vi "Create Notifiers.vi"(8 "error in":errorcluster) -> (0 "error out":errorcluster, 3 "Notifiers":T1)   [LabVIEW 2014]
uses:
  Notifiers.ctl
  Message Handler Loop Notifiers.ctl
  Hardware Control/Parameter Analyzer/Parameter Analyzer Notifiers.ctl
  Hardware Control/Switching Matrix/Switching Matrix Notifiers.ctl
  Hardware Control/Stress Control/StressControl Notifiers.ctl
  Hardware Control/Spectrometer/Spectrometer Notifiers.ctl
  Hardware Control/Switches and Mirrors/SwitchesMirrors Notifiers.ctl
  Hardware Control/Camera/Camera Notifiers.ctl
  Hardware Control/XYZ Stage/XYZ Notifications.ctl
  Hardware Control/Autofocus/Autofocus Notifiers.ctl
  Measurements/Optoelectronic Measurement/Optoelectronic Notifiers.ctl
  Measurements/Save Data/SaveData Notifiers.ctl
  Measurements/Instrument Sequence/Instrument Sequence Notifiers.ctl
panel:
  # "LICENSED MATERIALS – PROPERTY OF IBM\nCopyright IBM Corp. 2016,\nALL RIGHTS RESERVED"
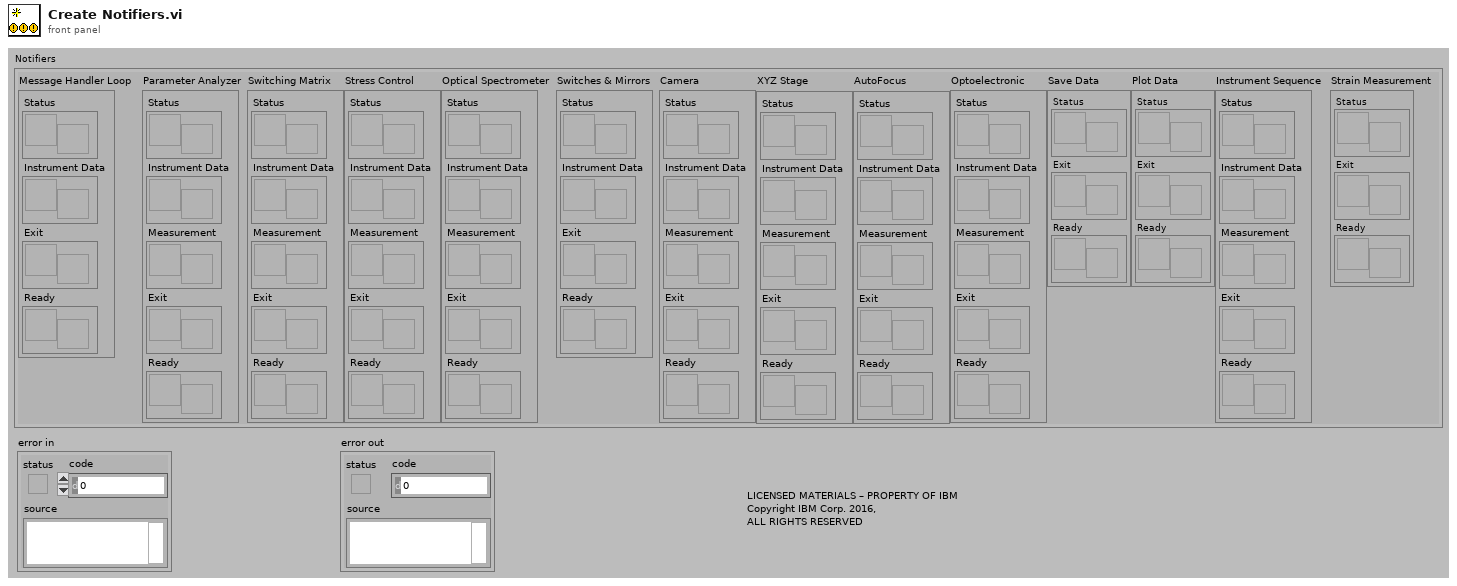
[diagram p1: front panel]
types:
  T1 = typedef "Notifiers.ctl" = cluster{"Message Handler Loop":T2, "Parameter Analyzer":T3, "Switching Matrix":T4, "Stress Control":T5, "Optical Spectrometer":T6, "Switches & Mirrors":T7, "Camera":T8, "XYZ Stage":T9, "AutoFocus":T10, "Optoelectronic":T11, "Save Data":T12, "Plot Data":T12, "Instrument Sequence":T13, "Strain Measurement":cluster{"Status":refnum<notifier>, "Exit":refnum<notifier>, "Ready":refnum<notifier>}}
  T2 = typedef "Message Handler Loop Notifiers.ctl" = cluster{"Status":refnum<notifier>, "Instrument Data":refnum<notifier>, "Exit":refnum<notifier>, "Ready":refnum<notifier>}
  T3 = typedef "Parameter Analyzer Notifiers.ctl" = cluster{"Status":refnum<notifier>, "Instrument Data":refnum<notifier>, "Measurement":refnum<notifier>, "Exit":refnum<notifier>, "Ready":refnum<notifier>}
  T4 = typedef "Switching Matrix Notifiers.ctl" = cluster{"Status":refnum<notifier>, "Instrument Data":refnum<notifier>, "Measurement":refnum<notifier>, "Exit":refnum<notifier>, "Ready":refnum<notifier>}
  T5 = typedef "StressControl Notifiers.ctl" = cluster{"Status":refnum<notifier>, "Instrument Data":refnum<notifier>, "Measurement":refnum<notifier>, "Exit":refnum<notifier>, "Ready":refnum<notifier>}
  T6 = typedef "Spectrometer Notifiers.ctl" = cluster{"Status":refnum<notifier>, "Instrument Data":refnum<notifier>, "Measurement":refnum<notifier>, "Exit":refnum<notifier>, "Ready":refnum<notifier>}
  T7 = typedef "SwitchesMirrors Notifiers.ctl" = cluster{"Status":refnum<notifier>, "Instrument Data":refnum<notifier>, "Exit":refnum<notifier>, "Ready":refnum<notifier>}
  T8 = typedef "Camera Notifiers.ctl" = cluster{"Status":refnum<notifier>, "Instrument Data":refnum<notifier>, "Measurement":refnum<notifier>, "Exit":refnum<notifier>, "Ready":refnum<notifier>}
  T9 = typedef "XYZ Notifications.ctl" = cluster{"Status":refnum<notifier>, "Instrument Data":refnum<notifier>, "Measurement":refnum<notifier>, "Exit":refnum<notifier>, "Ready":refnum<notifier>}
  T10 = typedef "Autofocus Notifiers.ctl" = cluster{"Status":refnum<notifier>, "Instrument Data":refnum<notifier>, "Measurement":refnum<notifier>, "Exit":refnum<notifier>, "Ready":refnum<notifier>}
  T11 = typedef "Optoelectronic Notifiers.ctl" = cluster{"Status":refnum<notifier>, "Instrument Data":refnum<notifier>, "Measurement":refnum<notifier>, "Exit":refnum<notifier>, "Ready":refnum<notifier>}
  T12 = typedef "SaveData Notifiers.ctl" = cluster{"Status":refnum<notifier>, "Exit":refnum<notifier>, "Ready":refnum<notifier>}
  T13 = typedef "Instrument Sequence Notifiers.ctl" = cluster{"Status":refnum<notifier>, "Instrument Data":refnum<notifier>, "Measurement":refnum<notifier>, "Exit":refnum<notifier>, "Ready":refnum<notifier>}
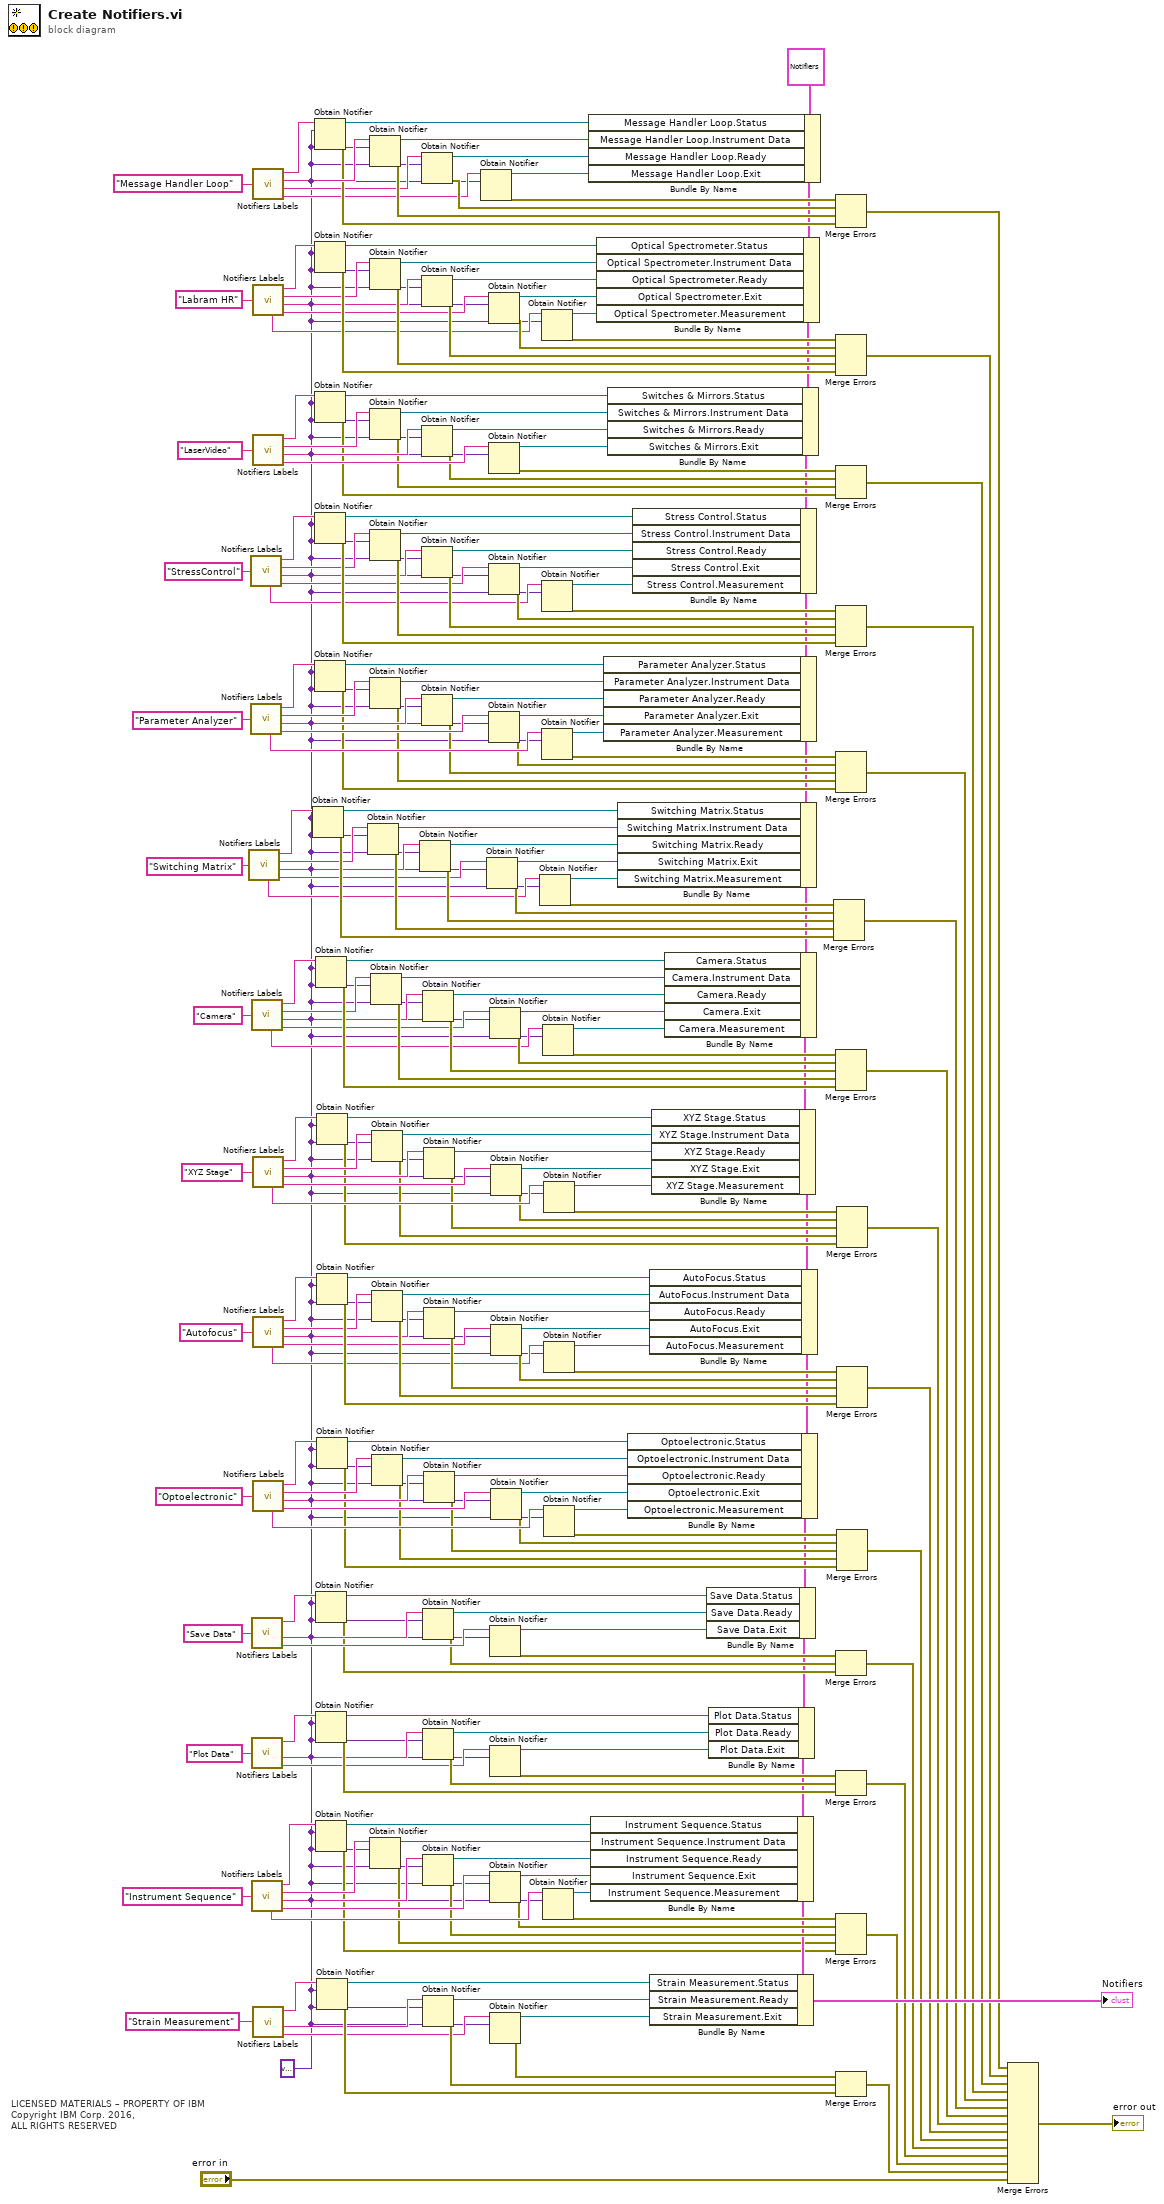
[diagram p0: block diagram]
diagram:
  w1 = variant ("element data type")
  # "LICENSED MATERIALS – PROPERTY OF IBM\nCopyright IBM Corp. 2016,\nALL RIGHTS RESERVED"
  n1 = call "Notifiers Labels.vi"("Instrument"="Switching Matrix") -> ("Exit String"=w117:string, "Ready String"=w118:string, "Data String"=w119:string, "Status String"=w120:string, "Measurement String"=w116:string)
  n2 = call "Notifiers Labels.vi"("Instrument"="StressControl") -> ("Exit String"=w185:string, "Ready String"=w186:string, "Data String"=w187:string, "Status String"=w188:string, "Measurement String"=w184:string)
  n3 = call "Notifiers Labels.vi"("Instrument"="Parameter Analyzer") -> ("Exit String"=w171:string, "Ready String"=w170:string, "Data String"=w169:string, "Status String"=w168:string, "Measurement String"=w172:string)
  n4 = call "Notifiers Labels.vi"("Instrument"="Camera") -> ("Exit String"=w148:string, "Ready String"=w149:string, "Data String"=w150:string, "Status String"=w151:string, "Measurement String"=w147:string)
  n5 = call "Notifiers Labels.vi"("Instrument"="Save Data") -> ("Exit String"=w104:string, "Ready String"=w103:string, "Status String"=w102:string)  [unwired: 2 out]
  n6 = call "Notifiers Labels.vi"("Instrument"="Plot Data") -> ("Exit String"=w70:string, "Ready String"=w71:string, "Status String"=w72:string)  [unwired: 2 out]
  n7 = call "Notifiers Labels.vi"("Instrument"="Instrument Sequence") -> ("Exit String"=w93:string, "Ready String"=w92:string, "Data String"=w86:string, "Status String"=w88:string, "Measurement String"=w94:string)
  n8 = call "Notifiers Labels.vi"("Instrument"="Message Handler Loop") -> ("Exit String"=w215:string, "Ready String"=w216:string, "Data String"=w228:string, "Status String"=w229:string)  [unwired: 1 out]
  n9 = call "Notifiers Labels.vi"("Instrument"="Labram HR") -> ("Exit String"=w204:string, "Ready String"=w205:string, "Data String"=w210:string, "Status String"=w211:string, "Measurement String"=w203:string)
  n10 = call "Notifiers Labels.vi"("Instrument"="LaserVideo") -> ("Exit String"=w201:string, "Ready String"=w200:string, "Data String"=w199:string, "Status String"=w198:string)  [unwired: 1 out]
  n11 = call "Notifiers Labels.vi"("Instrument"="XYZ Stage") -> ("Exit String"=w56:string, "Ready String"=w55:string, "Data String"=w54:string, "Status String"=w53:string, "Measurement String"=w57:string)
  n12 = call "Notifiers Labels.vi"("Instrument"="Autofocus") -> ("Exit String"=w39:string, "Ready String"=w40:string, "Data String"=w41:string, "Status String"=w42:string, "Measurement String"=w38:string)
  n13 = call "Notifiers Labels.vi"("Instrument"="Optoelectronic") -> ("Exit String"=w13:string, "Ready String"=w12:string, "Data String"=w11:string, "Status String"=w10:string, "Measurement String"=w14:string)
  n14 = call "Notifiers Labels.vi"("Instrument"="Strain Measurement") -> ("Exit String"=w77:string, "Ready String"=w76:string, "Status String"=w140:string)  [unwired: 2 out]
  n15 = Obtain Notifier(name (unnamed)=w120, notification data type=w1) -> (notifier out=w127:refnum<notifier>, error out=w121:errorcluster)  [unwired: 2 in, 1 out]
  n16 = Obtain Notifier(name (unnamed)=w229, notification data type=w1) -> (notifier out=w227:refnum<notifier>, error out=w225:errorcluster)  [unwired: 2 in, 1 out]
  n17 = Obtain Notifier(name (unnamed)=w211, notification data type=w1) -> (notifier out=w209:refnum<notifier>, error out=w213:errorcluster)  [unwired: 2 in, 1 out]
  n18 = Obtain Notifier(name (unnamed)=w198, notification data type=w1) -> (notifier out=w182:refnum<notifier>, error out=w197:errorcluster)  [unwired: 2 in, 1 out]
  n19 = Obtain Notifier(name (unnamed)=w188, notification data type=w1) -> (notifier out=w178:refnum<notifier>, error out=w189:errorcluster)  [unwired: 2 in, 1 out]
  n20 = Obtain Notifier(name (unnamed)=w168, notification data type=w1) -> (notifier out=w161:refnum<notifier>, error out=w167:errorcluster)  [unwired: 2 in, 1 out]
  n21 = Obtain Notifier(name (unnamed)=w151, notification data type=w1) -> (notifier out=w146:refnum<notifier>, error out=w152:errorcluster)  [unwired: 2 in, 1 out]
  n22 = Obtain Notifier(name (unnamed)=w102, notification data type=w1) -> (notifier out=w105:refnum<notifier>, error out=w99:errorcluster)  [unwired: 2 in, 1 out]
  n23 = Obtain Notifier(name (unnamed)=w72, notification data type=w1) -> (notifier out=w69:refnum<notifier>, error out=w75:errorcluster)  [unwired: 2 in, 1 out]
  n24 = Obtain Notifier(name (unnamed)=w88, notification data type=w1) -> (notifier out=w85:refnum<notifier>, error out=w83:errorcluster)  [unwired: 2 in, 1 out]
  n25 = Obtain Notifier(name (unnamed)=w53, notification data type=w1) -> (notifier out=w58:refnum<notifier>, error out=w52:errorcluster)  [unwired: 2 in, 1 out]
  n26 = Obtain Notifier(name (unnamed)=w42, notification data type=w1) -> (notifier out=w37:refnum<notifier>, error out=w43:errorcluster)  [unwired: 2 in, 1 out]
  n27 = Obtain Notifier(name (unnamed)=w10, notification data type=w1) -> (notifier out=w15:refnum<notifier>, error out=w9:errorcluster)  [unwired: 2 in, 1 out]
  n28 = Obtain Notifier(name (unnamed)=w140, notification data type=w1) -> (notifier out=w137:refnum<notifier>, error out=w139:errorcluster)  [unwired: 2 in, 1 out]
  n29 = Obtain Notifier(name (unnamed)=w119, notification data type=w1) -> (notifier out=w128:refnum<notifier>, error out=w125:errorcluster)  [unwired: 2 in, 1 out]
  n30 = Obtain Notifier(name (unnamed)=w228, notification data type=w1) -> (notifier out=w232:refnum<notifier>, error out=w224:errorcluster)  [unwired: 2 in, 1 out]
  n31 = Obtain Notifier(name (unnamed)=w210, notification data type=w1) -> (notifier out=w208:refnum<notifier>, error out=w222:errorcluster)  [unwired: 2 in, 1 out]
  n32 = Obtain Notifier(name (unnamed)=w199, notification data type=w1) -> (notifier out=w181:refnum<notifier>, error out=w194:errorcluster)  [unwired: 2 in, 1 out]
  n33 = Obtain Notifier(name (unnamed)=w187, notification data type=w1) -> (notifier out=w176:refnum<notifier>, error out=w193:errorcluster)  [unwired: 2 in, 1 out]
  n34 = Obtain Notifier(name (unnamed)=w169, notification data type=w1) -> (notifier out=w160:refnum<notifier>, error out=w163:errorcluster)  [unwired: 2 in, 1 out]
  n35 = Obtain Notifier(name (unnamed)=w86, notification data type=w1) -> (notifier out=w84:refnum<notifier>, error out=w82:errorcluster)  [unwired: 2 in, 1 out]
  n36 = Obtain Notifier(name (unnamed)=w150, notification data type=w1) -> (notifier out=w145:refnum<notifier>, error out=w156:errorcluster)  [unwired: 2 in, 1 out]
  n37 = Obtain Notifier(name (unnamed)=w54, notification data type=w1) -> (notifier out=w59:refnum<notifier>, error out=w48:errorcluster)  [unwired: 2 in, 1 out]
  n38 = Obtain Notifier(name (unnamed)=w41, notification data type=w1) -> (notifier out=w36:refnum<notifier>, error out=w47:errorcluster)  [unwired: 2 in, 1 out]
  n39 = Obtain Notifier(name (unnamed)=w11, notification data type=w1) -> (notifier out=w16:refnum<notifier>, error out=w5:errorcluster)  [unwired: 2 in, 1 out]
  n40 = Obtain Notifier(name (unnamed)=w118, notification data type=w1) -> (notifier out=w129:refnum<notifier>, error out=w124:errorcluster)  [unwired: 2 in, 1 out]
  n41 = Obtain Notifier(name (unnamed)=w216, notification data type=w1) -> (notifier out=w218:refnum<notifier>, error out=w223:errorcluster)  [unwired: 2 in, 1 out]
  n42 = Obtain Notifier(name (unnamed)=w205, notification data type=w1) -> (notifier out=w207:refnum<notifier>, error out=w221:errorcluster)  [unwired: 2 in, 1 out]
  n43 = Obtain Notifier(name (unnamed)=w200, notification data type=w1) -> (notifier out=w180:refnum<notifier>, error out=w195:errorcluster)  [unwired: 2 in, 1 out]
  n44 = Obtain Notifier(name (unnamed)=w186, notification data type=w1) -> (notifier out=w175:refnum<notifier>, error out=w192:errorcluster)  [unwired: 2 in, 1 out]
  n45 = Obtain Notifier(name (unnamed)=w170, notification data type=w1) -> (notifier out=w159:refnum<notifier>, error out=w164:errorcluster)  [unwired: 2 in, 1 out]
  n46 = Obtain Notifier(name (unnamed)=w149, notification data type=w1) -> (notifier out=w144:refnum<notifier>, error out=w155:errorcluster)  [unwired: 2 in, 1 out]
  n47 = Obtain Notifier(name (unnamed)=w103, notification data type=w1) -> (notifier out=w106:refnum<notifier>, error out=w100:errorcluster)  [unwired: 2 in, 1 out]
  n48 = Obtain Notifier(name (unnamed)=w71, notification data type=w1) -> (notifier out=w68:refnum<notifier>, error out=w74:errorcluster)  [unwired: 2 in, 1 out]
  n49 = Obtain Notifier(name (unnamed)=w92, notification data type=w1) -> (notifier out=w95:refnum<notifier>, error out=w89:errorcluster)  [unwired: 2 in, 1 out]
  n50 = Obtain Notifier(name (unnamed)=w76, notification data type=w1) -> (notifier out=w78:refnum<notifier>, error out=w80:errorcluster)  [unwired: 2 in, 1 out]
  n51 = Obtain Notifier(name (unnamed)=w55, notification data type=w1) -> (notifier out=w60:refnum<notifier>, error out=w49:errorcluster)  [unwired: 2 in, 1 out]
  n52 = Obtain Notifier(name (unnamed)=w40, notification data type=w1) -> (notifier out=w35:refnum<notifier>, error out=w46:errorcluster)  [unwired: 2 in, 1 out]
  n53 = Obtain Notifier(name (unnamed)=w12, notification data type=w1) -> (notifier out=w17:refnum<notifier>, error out=w6:errorcluster)  [unwired: 2 in, 1 out]
  n54 = Obtain Notifier(name (unnamed)=w215, notification data type=w1) -> (notifier out=w217:refnum<notifier>, error out=w214:errorcluster)  [unwired: 2 in, 1 out]
  n55 = Obtain Notifier(name (unnamed)=w117, notification data type=w1) -> (notifier out=w130:refnum<notifier>, error out=w123:errorcluster)  [unwired: 2 in, 1 out]
  n56 = Obtain Notifier(name (unnamed)=w204, notification data type=w1) -> (notifier out=w206:refnum<notifier>, error out=w220:errorcluster)  [unwired: 2 in, 1 out]
  n57 = Obtain Notifier(name (unnamed)=w201, notification data type=w1) -> (notifier out=w179:refnum<notifier>, error out=w196:errorcluster)  [unwired: 2 in, 1 out]
  n58 = Obtain Notifier(name (unnamed)=w185, notification data type=w1) -> (notifier out=w174:refnum<notifier>, error out=w191:errorcluster)  [unwired: 2 in, 1 out]
  n59 = Obtain Notifier(name (unnamed)=w171, notification data type=w1) -> (notifier out=w158:refnum<notifier>, error out=w165:errorcluster)  [unwired: 2 in, 1 out]
  n60 = Obtain Notifier(name (unnamed)=w148, notification data type=w1) -> (notifier out=w143:refnum<notifier>, error out=w154:errorcluster)  [unwired: 2 in, 1 out]
  n61 = Obtain Notifier(name (unnamed)=w104, notification data type=w1) -> (notifier out=w107:refnum<notifier>, error out=w101:errorcluster)  [unwired: 2 in, 1 out]
  n62 = Obtain Notifier(name (unnamed)=w70, notification data type=w1) -> (notifier out=w67:refnum<notifier>, error out=w73:errorcluster)  [unwired: 2 in, 1 out]
  n63 = Obtain Notifier(name (unnamed)=w93, notification data type=w1) -> (notifier out=w96:refnum<notifier>, error out=w90:errorcluster)  [unwired: 2 in, 1 out]
  n64 = Obtain Notifier(name (unnamed)=w77, notification data type=w1) -> (notifier out=w81:refnum<notifier>, error out=w79:errorcluster)  [unwired: 2 in, 1 out]
  n65 = Obtain Notifier(name (unnamed)=w56, notification data type=w1) -> (notifier out=w61:refnum<notifier>, error out=w50:errorcluster)  [unwired: 2 in, 1 out]
  n66 = Obtain Notifier(name (unnamed)=w39, notification data type=w1) -> (notifier out=w34:refnum<notifier>, error out=w45:errorcluster)  [unwired: 2 in, 1 out]
  n67 = Obtain Notifier(name (unnamed)=w13, notification data type=w1) -> (notifier out=w18:refnum<notifier>, error out=w7:errorcluster)  [unwired: 2 in, 1 out]
  n68 = Obtain Notifier(name (unnamed)=w116, notification data type=w1) -> (notifier out=w131:refnum<notifier>, error out=w122:errorcluster)  [unwired: 2 in, 1 out]
  n69 = Obtain Notifier(name (unnamed)=w203, notification data type=w1) -> (notifier out=w202:refnum<notifier>, error out=w219:errorcluster)  [unwired: 2 in, 1 out]
  n70 = Obtain Notifier(name (unnamed)=w184, notification data type=w1) -> (notifier out=w173:refnum<notifier>, error out=w190:errorcluster)  [unwired: 2 in, 1 out]
  n71 = Obtain Notifier(name (unnamed)=w172, notification data type=w1) -> (notifier out=w157:refnum<notifier>, error out=w166:errorcluster)  [unwired: 2 in, 1 out]
  n72 = Obtain Notifier(name (unnamed)=w147, notification data type=w1) -> (notifier out=w142:refnum<notifier>, error out=w153:errorcluster)  [unwired: 2 in, 1 out]
  n73 = Obtain Notifier(name (unnamed)=w94, notification data type=w1) -> (notifier out=w97:refnum<notifier>, error out=w91:errorcluster)  [unwired: 2 in, 1 out]
  n74 = Obtain Notifier(name (unnamed)=w57, notification data type=w1) -> (notifier out=w62:refnum<notifier>, error out=w51:errorcluster)  [unwired: 2 in, 1 out]
  n75 = Obtain Notifier(name (unnamed)=w38, notification data type=w1) -> (notifier out=w33:refnum<notifier>, error out=w44:errorcluster)  [unwired: 2 in, 1 out]
  n76 = Obtain Notifier(name (unnamed)=w14, notification data type=w1) -> (notifier out=w19:refnum<notifier>, error out=w8:errorcluster)  [unwired: 2 in, 1 out]
  n77 = Bundle By Name(cluster=T1 {"Message Handler Loop"={"Status"=refnum, "Instrument Data"=refnum, "Exit"=refnum, "Ready"=refnum}, "Parameter Analyzer"={"Status"=refnum, "Instrument Data"=refnum, "Measurement"=refnum, "Exit"=refnum, "Ready"=refnum}, "Switching Matrix"={"Status"=refnum, "Instrument Data"=refnum, "Measurement"=refnum, "Exit"=refnum, "Ready"=refnum}, "Stress Control"={"Status"=refnum, "Instrument Data"=refnum, "Measurement"=refnum, "Exit"=refnum, "Ready"=refnum}, "Optical Spectrometer"={"Status"=refnum, "Instrument Data"=refnum, "Measurement"=refnum, "Exit"=refnum, "Ready"=refnum}, "Switches & Mirrors"={"Status"=refnum, "Instrument Data"=refnum, "Exit"=refnum, "Ready"=refnum}, "Camera"={"Status"=refnum, "Instrument Data"=refnum, "Measurement"=refnum, "Exit"=refnum, "Ready"=refnum}, "XYZ Stage"={"Status"=refnum, "Instrument Data"=refnum, "Measurement"=refnum, "Exit"=refnum, "Ready"=refnum}, "AutoFocus"={"Status"=refnum, "Instrument Data"=refnum, "Measurement"=refnum, "Exit"=refnum, "Ready"=refnum}, "Optoelectronic"={"Status"=refnum, "Instrument Data"=refnum, "Measurement"=refnum, "Exit"=refnum, "Ready"=refnum}, "Save Data"={"Status"=refnum, "Exit"=refnum, "Ready"=refnum}, "Plot Data"={"Status"=refnum, "Exit"=refnum, "Ready"=refnum}, "Instrument Sequence"={"Status"=refnum, "Instrument Data"=refnum, "Measurement"=refnum, "Exit"=refnum, "Ready"=refnum}, "Strain Measurement"={"Status"=refnum, "Exit"=refnum, "Ready"=refnum}} ("Notifiers 2"), "Message Handler Loop.Status"=w227, "Message Handler Loop.Instrument Data"=w232, "Message Handler Loop.Ready"=w218, "Message Handler Loop.Exit"=w217) -> (w114:T1)
  n78 = Bundle By Name(cluster=w114, "Optical Spectrometer.Status"=w209, "Optical Spectrometer.Instrument Data"=w208, "Optical Spectrometer.Ready"=w207, "Optical Spectrometer.Exit"=w206, "Optical Spectrometer.Measurement"=w202) -> (w113:T1)
  n79 = Bundle By Name(cluster=w113, "Switches & Mirrors.Status"=w182, "Switches & Mirrors.Instrument Data"=w181, "Switches & Mirrors.Ready"=w180, "Switches & Mirrors.Exit"=w179) -> (w112:T1)
  n80 = Bundle By Name(cluster=w112, "Stress Control.Status"=w178, "Stress Control.Instrument Data"=w176, "Stress Control.Ready"=w175, "Stress Control.Exit"=w174, "Stress Control.Measurement"=w173) -> (w111:T1)
  n81 = Bundle By Name(cluster=w111, "Parameter Analyzer.Status"=w161, "Parameter Analyzer.Instrument Data"=w160, "Parameter Analyzer.Ready"=w159, "Parameter Analyzer.Exit"=w158, "Parameter Analyzer.Measurement"=w157) -> (w110:T1)
  n82 = Bundle By Name(cluster=w110, "Switching Matrix.Status"=w127, "Switching Matrix.Instrument Data"=w128, "Switching Matrix.Ready"=w129, "Switching Matrix.Exit"=w130, "Switching Matrix.Measurement"=w131) -> (w109:T1)
  n83 = Bundle By Name(cluster=w109, "Camera.Status"=w146, "Camera.Instrument Data"=w145, "Camera.Ready"=w144, "Camera.Exit"=w143, "Camera.Measurement"=w142) -> (w31:T1)
  n84 = Bundle By Name(cluster=w31, "XYZ Stage.Status"=w58, "XYZ Stage.Instrument Data"=w59, "XYZ Stage.Ready"=w60, "XYZ Stage.Exit"=w61, "XYZ Stage.Measurement"=w62) -> (w30:T1)
  n85 = Bundle By Name(cluster=w30, "AutoFocus.Status"=w37, "AutoFocus.Instrument Data"=w36, "AutoFocus.Ready"=w35, "AutoFocus.Exit"=w34, "AutoFocus.Measurement"=w33) -> (w4:T1)
  n86 = Bundle By Name(cluster=w4, "Optoelectronic.Status"=w15, "Optoelectronic.Instrument Data"=w16, "Optoelectronic.Ready"=w17, "Optoelectronic.Exit"=w18, "Optoelectronic.Measurement"=w19) -> (w3:T1)
  n87 = Bundle By Name(cluster=w3, "Save Data.Status"=w105, "Save Data.Ready"=w106, "Save Data.Exit"=w107) -> (w65:T1)
  n88 = Bundle By Name(cluster=w65, "Plot Data.Status"=w69, "Plot Data.Ready"=w68, "Plot Data.Exit"=w67) -> (w64:T1)
  n89 = Bundle By Name(cluster=w64, "Instrument Sequence.Status"=w85, "Instrument Sequence.Instrument Data"=w84, "Instrument Sequence.Ready"=w95, "Instrument Sequence.Exit"=w96, "Instrument Sequence.Measurement"=w97) -> (w87:T1)
  n90 = Bundle By Name(cluster=w87, "Strain Measurement.Status"=w137, "Strain Measurement.Ready"=w78, "Strain Measurement.Exit"=w81) -> (→"Notifiers":T1)
  n91 = Merge Errors(w122, w123, w124, w125, w121) -> (w115:errorcluster)
  n92 = Merge Errors(w214, w223, w224, w225) -> (w132:errorcluster)
  n93 = Merge Errors(w219, w220, w221, w222, w213) -> (w133:errorcluster)
  n94 = Merge Errors(w196, w195, w194, w197) -> (w134:errorcluster)
  n95 = Merge Errors(w190, w191, w192, w193, w189) -> (w135:errorcluster)
  n96 = Merge Errors(w166, w165, w164, w163, w167) -> (w136:errorcluster)
  n97 = Merge Errors(w153, w154, w155, w156, w152) -> (w26:errorcluster)
  n98 = Merge Errors(w101, w100, w99) -> (w27:errorcluster)
  n99 = Merge Errors(w73, w74, w75) -> (w28:errorcluster)
  n100 = Merge Errors(w91, w90, w89, w82, w83) -> (w29:errorcluster)
  n101 = Merge Errors(w79, w80, w139) -> (w23:errorcluster)
  n102 = Merge Errors(w51, w50, w49, w48, w52) -> (w24:errorcluster)
  n103 = Merge Errors(w44, w45, w46, w47, w43) -> (w25:errorcluster)
  n104 = Merge Errors(w8, w7, w6, w5, w9) -> (w2:errorcluster)
  n105 = Merge Errors(w132, w133, w134, w135, w136, w115, w26, w24, w25, w2, w27, w28, w29, w23, "error in") -> (→"error out":errorcluster)
